vi "Upd Desired Gas.vi"(8 "error in (no error)":errorcluster, 10 "Desired Gas":string, 11 "C100L in":refnum<class "C100L.lvclass">) -> (0 "error out":errorcluster, 3 "C100L out":refnum<class "C100L.lvclass">)   [LabVIEW 2021, in "C100L.lvlib" / "C100L.lvclass"]
uses:
  C100L.lvclass
  C100L.lvclass/C100L.ctl
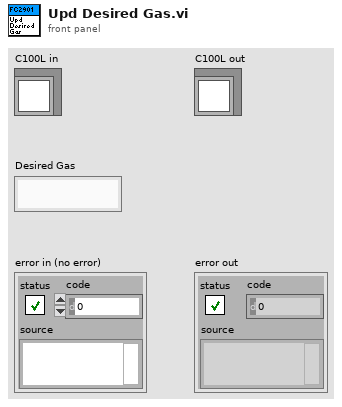
[diagram p1: front panel]
types:
  T1 = typedef "C100L.lvlib/C100L.lvclass/GCF Data.ctl" = map{string, dbl}
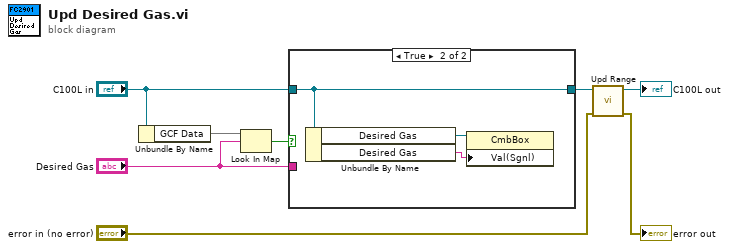
[diagram p0: block diagram]
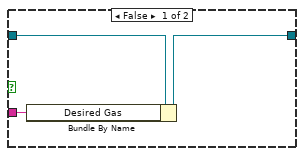
[diagram p2: hidden frame]
diagram:
  n1 = Unbundle By Name("C100L in") -> ("GCF Data"=w5:T1)
  n2 = Look In Map(map=w5, key="Desired Gas") -> (key not found?=w4:bool)  [unwired: 1 in, 1 out]
  n3 = case shown="True" w4 {
    tunnel: "C100L in" -> [w11 w12]
    tunnel: [w10 w12] -> w2
    tunnel: "Desired Gas" -> [w9 _]
    frame False {
      n4 = Bundle By Name(cluster=w11, "Desired Gas"=w9) -> (w10:refnum<class "C100L.lvclass">)
    }
    frame True {
      n5 = Unbundle By Name(w12) -> ("Desired Gas"=w14:refnum<vi>, "Desired Gas"=w13:string)
      n6 = property class="CmbBox"(reference=w14, "Val(Sgnl)"=w13) -> ()  [unwired: 1 in, 2 out]
    }
  }
  n7 = call "Upd Range.vi"("error in (no error)"="error in (no error)", "C100L in"=w2) -> ("error out"=→"error out":errorcluster, "C100L out"=→"C100L out":refnum<class "C100L.lvclass">)  [unwired: 8 in]
